vi "Edit Current Error code.vi"(9 "VI Path":path=path "C:/GitClones/PantherDashboard/src/LabVIEW/Test Project/Errors/ProjectERR--error.vi", 11 "Error Codes and Descriptions":string[][](array[string])) -> (3 "Refresh":bool)   [LabVIEW 2020, in "ConstantErrorsMaker.lvlib"]
uses:
  ConstantErrorsMaker.lvlib
  <vilib>/Utility/traverseref.llb/TRef TravTarget.ctl
panel:
  in  "Cancel":bool
  in  "Continue":bool
  in  "Current error code (0)":i32=5001
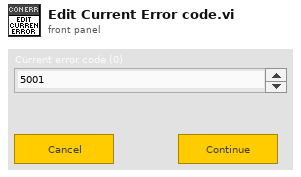
[diagram p1: front panel]
types:
  T1 = typedef "TRef TravTarget.ctl" = enum16{"FP", "BD", "Other"}
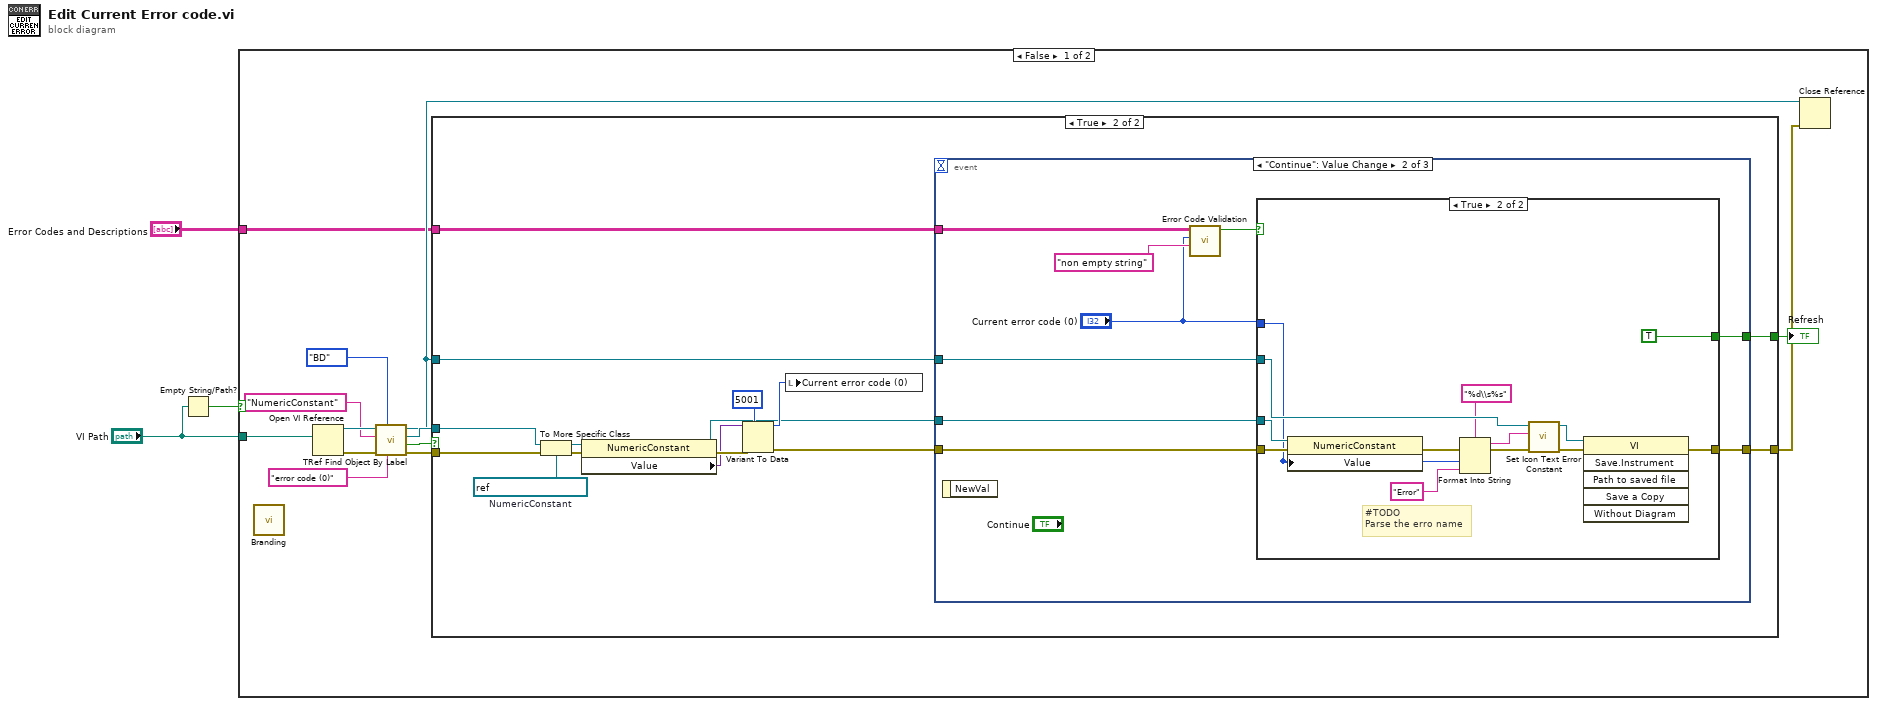
[diagram p0: block diagram]
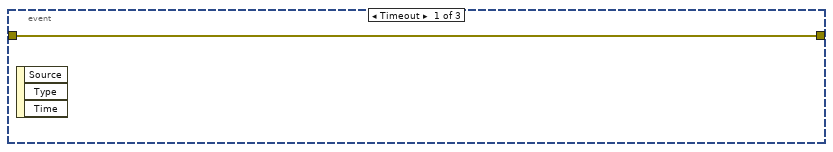
[diagram p3: hidden frame]
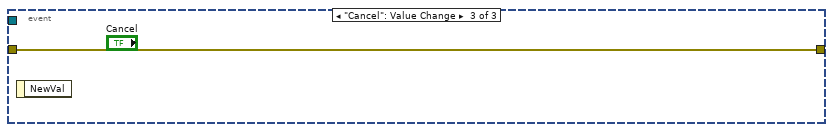
[diagram p5: hidden frame]
diagram:
  n1 = Empty String/Path?(string/path="VI Path") -> (empty?=w1:bool)
  n2 = case shown="False" w1 {
    tunnel: "Error Codes and Descriptions" -> [w6 _]
    tunnel: "VI Path" -> [w5 _]
    frame False {
      n3 = call "Branding.vi"() -> ()  [unwired: 12 in]
      n4 = Open VI Reference(vi path=w5) -> (vi reference=w13:refnum<vi>, error out=w16:errorcluster)  [unwired: 5 in]
      n5 = call <vilib>:"TRef Find Object By Label.vi"("Label"="error code (0)", "Traverse Target"=TRef_TravTarget."BD", "error in (no error)"=w16, "Class Name"="NumericConstant", "VI Ref"=w13) -> ("error out"=w15:errorcluster, "Found?"=w8:bool, "Found Obj Ref"=w9:refnum<vi>, "dup VI Ref"=w7:refnum<vi>)  [unwired: 3 in]
      n6 = case shown="True" w8 {
        tunnel: w15 -> [w17 w32]
        tunnel: w9 -> [_ w27]
        tunnel: [w17 w28] -> w14
        tunnel: w7 -> [_ w20]
        tunnel: w6 -> [_ w19]
        tunnel: [_ w18] -> w4
        frame False {
        }
        frame True {
          w26 = refnum<vi> refnum  # NumericConstant
          n7 = To More Specific Class(target class=w26, reference=w27, error in=w32) -> (specific class reference=w25:refnum<vi>, error out=w31:errorcluster)
          n8 = property class="NumericConstant"(reference=w25, error in=w31) -> (reference out=w21:refnum<vi>, error out=w30:errorcluster, "Value"=w23:variant)
          n9 = Variant To Data(error in=w30, type=5001 ("error code (0)"), Variant=w23) -> (data=w22:i32, error out=w29:errorcluster)
          n10 = local write "Current error code (0)"(w22) -> ()
          n11 = event shown="[1] \"Continue\": Value Change" {
            selector: _ -> [_ _ _]
            dyn-events: _ -> [_ _ _]
            timeout: _ -> [_ _ _]
            tunnel: w21 -> [_ w40 _]
            tunnel: [w33 w41 w56] -> w28
            tunnel: w29 -> [w33 w42 w56]
            tunnel: w20 -> [_ w38 _]
            tunnel: w19 -> [_ w37 _]
            tunnel: [_ w34 _] -> w18
            event Timeout {
              n12 = event-data() -> ()  [unwired: 1 in, 3 out]
            }
            event "Continue": Value Change {
              n13 = event-data() -> ()  [unwired: 1 in, 1 out]
              n14 = call "Error Code Validation.vi"("Error Name"="non empty string", "New Error Code"="Current error code (0)", "Error Codes and Descriptions"=w37) -> ("Continue"=w39:bool)  [unwired: 8 in]
              n15 = case shown="True" w39 {
                tunnel: w42 -> [w43 w55]
                tunnel: w40 -> [_ w51]
                tunnel: [w43 w52] -> w41
                tunnel: "Current error code (0)" -> [_ w48]
                tunnel: w38 -> [_ w50]
                tunnel: [_ TRUE] -> w34
                frame False {
                }
                frame True {
                  # "#TODO\nParse the erro name"
                  n16 = property class="NumericConstant"(reference=w51, error in=w55, "Value"=w48) -> (error out=w54:errorcluster)  [unwired: 1 out]
                  n17 = Format Into String(format string="%d\\s%s", w48, "Error" ("input 2")) -> (resulting string=w47:string)  [unwired: 2 in, 1 out]
                  n18 = call "Set Icon Text Error Constant.vi"("error in"=w54, "Text"=w47, "VI in"=w50) -> ("error out"=w53:errorcluster, "VI out"=w46:refnum<vi>)  [unwired: 7 in]
                  n19 = invoke class="VI" method="Save.Instrument"(reference=w46, error in=w53) -> (error out=w52:errorcluster)  [unwired: 4 in, 5 out]
                }
              }
            }
            event "Cancel": Value Change {
              n20 = event-data() -> ()  [unwired: 1 in, 1 out]
            }
          }
        }
      }
      "Refresh" <- w4
      n21 = Close Reference(reference=w7, error in (no error)=w14) -> ()  [unwired: 1 out]
    }
    frame True {
    }
  }
